vi "Write.vi"(8 "error in (no error)":errorcluster, 9 "Data":u8[](array[numeric]) format="%.0x", 10 "Address":u8 format="%.0x", 11 "I2C Bus In":refnum<class "I2C Bus.lvclass">) -> (0 "error out":errorcluster, 3 "I2C Bus Out":refnum<class "I2C Bus.lvclass">)   [LabVIEW 2020, in "I2C Bus.lvclass"]
uses:
  I2C Bus.lvclass
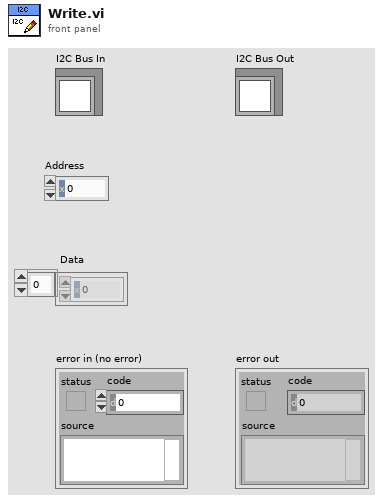
[diagram p1: front panel]
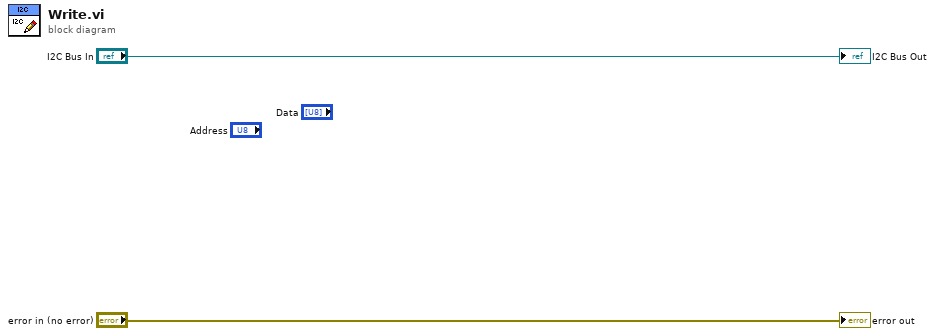
[diagram p0: block diagram]
diagram:
  "error out" <- "error in (no error)"
  "I2C Bus Out" <- "I2C Bus In"
